vi "SVL Restore Waterfall Window.vi"(0 "waterfall ref":refnum<vi>, 11 "error in (no error)":errorcluster, 12 "frontmost (T)":bool=TRUE) -> (4 "dup waterfall ref":refnum<vi>, 15 "error out":errorcluster)   [LabVIEW 2017]
doc: "Restores any existing waterfall window you unintentionally closed."
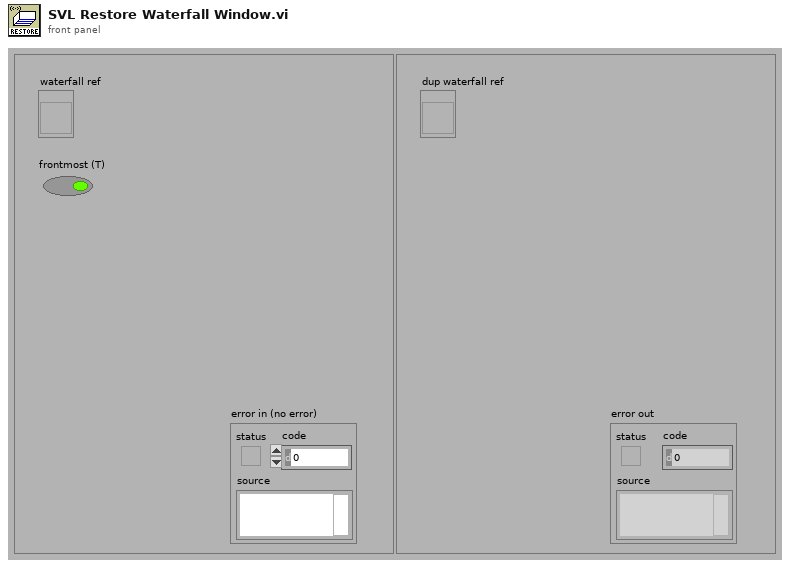
[diagram p1: front panel]
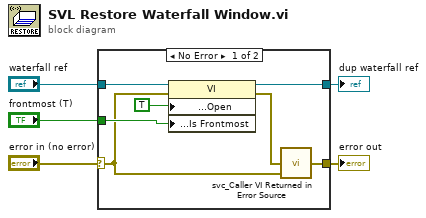
[diagram p0: block diagram]
diagram:
  n1 = case shown="No Error" "error in (no error)" {
    selector: "error in (no error)" -> [w6 w14]
    tunnel: [w12 w13] -> w5
    tunnel: "waterfall ref" -> [w11 w13]
    tunnel: "frontmost (T)" -> [w10 _]
    tunnel: [w7 w14] -> w2
    frame No Error {
      n2 = property class="VI"(reference=w11, error in=w6, "Front Panel Window:Open"=TRUE ("Front Panel.IsFrontmost"), "Front Panel Window:Is Frontmost"=w10) -> (reference out=w12:refnum<vi>, error out=w8:errorcluster)
      n3 = call <vilib>:"svc_Caller VI Returned in Error Source.vi"("warning input to caller"=w6, "error in (no error)"=w8) -> ("error out"=w7:errorcluster)  [unwired: 3 in]
    }
    frame Error {
    }
  }
  "dup waterfall ref" <- w5
  "error out" <- w2
